vi "MSScript_Calc_ArrayDiv.vi"(5 "VarString in":string, 6 "Value Error?":bool[](array[boolean]), 7 "Split Index":i32[](array[numeric]), 8 "ArrayVariable in":ext[](array[numeric]), 9 "Param Items":i32) -> (0 "ArrayVariable out":ext[](array[numeric]), 2 "CmdError?":bool)   [LabVIEW 2018, in "MSScript.lvclass"]
uses:
  MSScript.lvclass
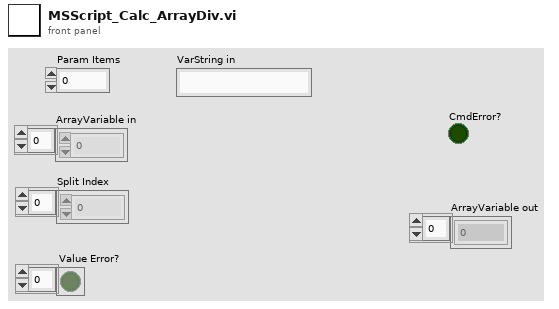
[diagram p1: front panel]
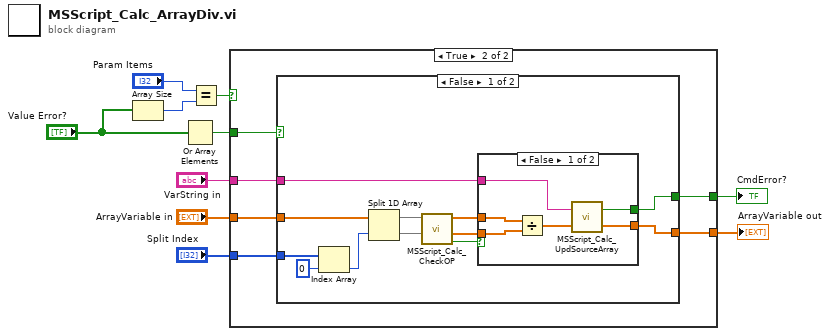
[diagram p0: block diagram]
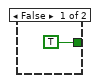
[diagram p2: hidden frame]
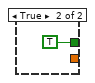
[diagram p3: hidden frame]
diagram:
  n1 = Array Size(array="Value Error?") -> (size(s)=w7:i32)
  n2 = Or Array Elements(Boolean array="Value Error?") -> (logical OR=w9:bool)
  n3 = Equal?(x="Param Items", y=w7) -> (x = y?=w5:bool)
  n4 = case shown="True" w5 {
    tunnel: [TRUE w12] -> w4
    tunnel: w9 -> [_ w17]
    tunnel: [_ w13] -> w10
    tunnel: "VarString in" -> [_ w16]
    tunnel: "ArrayVariable in" -> [_ w15]
    tunnel: "Split Index" -> [_ w14]
    frame False {
    }
    frame True {
      n5 = case shown="False" w17 {
        tunnel: w15 -> [w26 _]
        tunnel: [w24 _] -> w13
        tunnel: w14 -> [w27 _]
        tunnel: [w23 _] -> w12
        tunnel: w16 -> [w18 _]
        frame False {
          n6 = Index Array(array=w27, index=0) -> (element=w28:i32)
          n7 = Split 1D Array(array=w26, index=w28) -> (first subarray=w21:ext[], second subarray=w22:ext[])
          n8 = call "MSScript_Calc_CheckOP.vi"("Operator in"=w22, "Operand in"=w21) -> ("Cmd Error?"=w25:bool, "Operator out"=w19:ext[], "Operand out"=w20:ext[])  [unwired: 3 in]
          n9 = case shown="False" w25 {
            tunnel: [w34 _] -> w24
            tunnel: [w35 TRUE ("Value Error?")] -> w23
            tunnel: w20 -> [w31 _]
            tunnel: w19 -> [w32 _]
            tunnel: w18 -> [w30 _]
            frame False {
              n10 = Divide(x=w31, y=w32) -> (x/y=w33:ext[])
              n11 = call "MSScript_Calc_UpdSourceArray.vi"("ArrayVariable in"=w33, "VarString in"=w30) -> ("ArrayVariable out"=w34:ext[], "Cmd Error?"=w35:bool)
            }
            frame True {
            }
          }
        }
        frame True {
        }
      }
    }
  }
  "ArrayVariable out" <- w10
  "CmdError?" <- w4
